vi "移位寄存器1.vi"() -> ()   [LabVIEW 2023]
panel:
  out "example 3":i32
  out "example 2":i32
  out "example 1":i32
  # "这个东西 很导人。。。 巴嘎"
  # "移位寄存器"
  # "有文本编程语言经验的用户，刚开始接触 LabVIEW 时，遇到需要传递数据的情况，往往会先考虑创建一个变量，用变量来传递数据。在使用循环语句时，更是如此。\n这实际上是与 LabVIEW 的数据流驱动相违背的。使用 LabVIEW 的时候，需要转换思路，凡是循环内需要使用变量的地方，首先应考虑使用移位寄存器。"
  # "通过移位寄存器传入传出数据，数据的类型和值都不会发生变化。移位寄存器的特殊之处在于，在循环结构两端的接线端是强制使用同一内存的。\n因此，上一次迭代执行产生的某个数据，传给移位寄存器右侧的接线端，如果下一次迭代运行需要用到这个数据，从移位寄存器左侧的接线端引出就可以了。\n也就是说，尽管一对移位寄存器总是包含左右两部分，但这两部分中的数据是同一份；而隧道则有输入隧道和输出隧道之分，某个输入隧道是与其它输出隧道毫无关系的独立节点。"
  # "使用循环结构的一个常见错误是忘记给移位寄存器赋一个初始值。因此，\n使用移位寄存器时要切记：在循环结构外，给移位寄存器左侧端传入一个初始值，除非能够确定程序的确不需要给移位寄存器赋初值。"
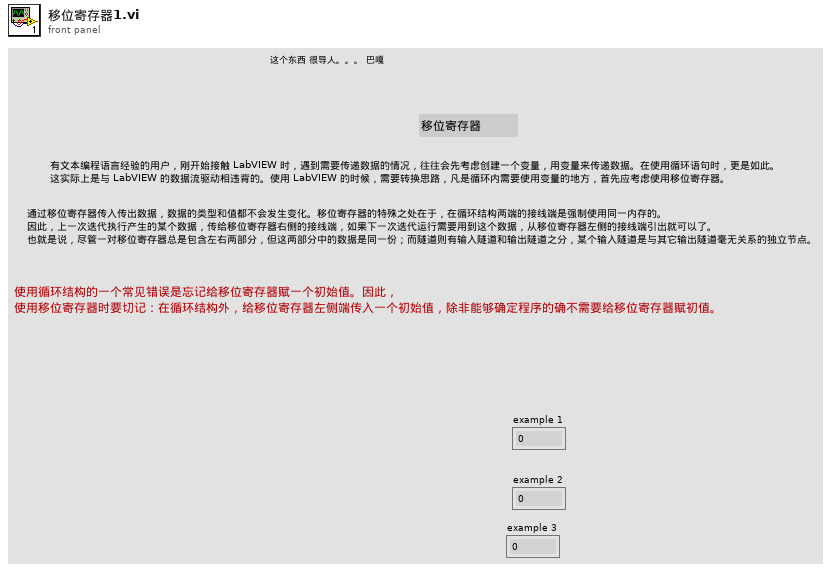
[diagram p1: front panel]
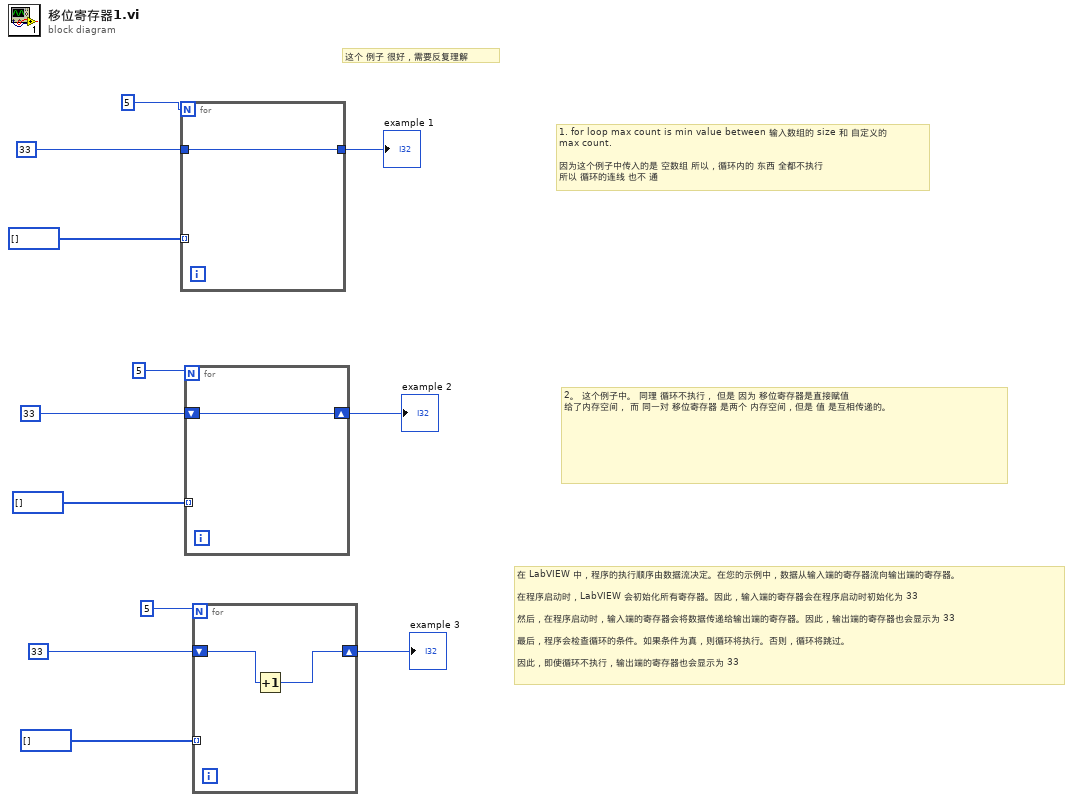
[diagram p0: block diagram]
diagram:
  # "在 LabVIEW 中，程序的执行顺序由数据流决定。在您的示例中，数据从输入端的寄存器流向输出端的寄存器。\n\n在程序启动时，LabVIEW 会初始化所有寄存器。因此，输入端的寄存器会在程序启动时初始化为 33\n\n然后，在程序启动时，输入端的寄存器会将数据传递给输出端的寄存器。因此，输出端的寄存器也会显示为 33\n\n最后，程序会检查循环的条件。如果条件为真，则循环将执行。否则，循环将跳过。\n\n因此，即使循环不执行，输出端的寄存器也会显示为 33"
  # "这个 例子 很好，需要反复理解"
  # "2。 这个例子中。 同理 循环不执行， 但是 因为 移位寄存器是直接赋值\n给了内存空间， 而 同一对 移位寄存器 是两个 内存空间，但是 值 是互相传递的。"
  # "1. for loop max count is min value between 输入数组的 size 和 自定义的\nmax count.\n\n因为这个例子中传入的是 空数组 所以，循环内的 东西 全都不执行\n所以 循环的连线 也不 通"
  n1 = for {
    N: 5 -> [_]
    tunnel: 33 -> [w13]
    tunnel: [w13] -> w11
    tunnel: i32[] [] -> [_] mode=indexing
  }
  "example 1" <- w11
  n2 = for {
    N: 5 -> [_]
    tunnel: i32[] [] -> [_] mode=indexing
    shift-right: [w14] -> w7
    shift-left: 33 -> [w14]
  }
  "example 2" <- w7
  n3 = for {
    N: 5 -> [_]
    tunnel: i32[] [] -> [_] mode=indexing
    shift-right: [w15] -> w2
    shift-left: 33 -> [w16]
    n4 = Increment(x=w16) -> (x+1=w15:i32)
  }
  "example 3" <- w2
